vi "myRIO_BRig_FPGA_v3,3.vi"() -> ()   [LabVIEW 2014]
uses:
  <vilib>/rvi/FXPMathLib/FxpDiv/subVIs/nifxpmath_Div_SimConfig.ctl
  <vilib>/rvi/FXPMathLib/FxpSinAndCos/subVIs/nifxpmath_SinAndCos_SimConfig.ctl
  <vilib>/rvi/FXPMathLib/FxpDiv/simVIs/DllFxpDivTemp_sub.vi
  <vilib>/rvi/FXPMathLib/FxpSinAndCos/simVIs/DllFxpSinAndCosTemp_sub.vi
  <vilib>/rvi/Emulation/niFpgaGetClockAttributes.vi
  <vilib>/rvi/Emulation/niFpgaSctlEmulationGetInTimedLoop.vi
  <vilib>/rvi/Emulation/niFpgaEmulationReportErrorSimple.vi
  <vilib>/rvi/eio/common/nirviEmuTemplateMethod_errors.vi
  <vilib>/rvi/Emulation/niFpgaCriticalErrorInLSC.vi
  <vilib>/rvi/FXPMathLib/FxpDiv/XNode/nifxpmath_Div.xnode
  <vilib>/rvi/FXPMathLib/FxpMul/XNode/nifxpmath_Multiplier.xnode
  <vilib>/rvi/FXPMathLib/FxpSinAndCos/XNode/nifxpmath_SinAndCos.xnode
  <vilib>/rvi/FXPMathLib/FxpSub/XNode/nifxpmath_Sub.xnode
  <vilib>/eio/EIONode/EIONode.xnode
  <vilib>/rvi/FXPMathLib/sim/FxpSim.dll
panel:
  in  "laser_Nshutter":u32=100
  in  "AnaOut_0":u16
  in  "f_time_select":u32=173
  in  "laser_Nvalley":u32=100
  in  "laser_Npeak":u32=100
  in  "laserledMTrig":bool
  in  "tCycle_laser_wro":u32=100
  in  "tDelay_laser_wro":u32
  in  "tCycle_laser_rew":u32=100
  in  "tDelay_laser_rew":u32
  in  "laserResponse_reward_LED":bool
  in  "laserResponse_wrong_LED":bool
  out "SelectWrong":bool
  out "SelectReward":bool
  in  "laserResponse_wrong":bool
  in  "laserResponse_reward":bool
  in  "Left(F)_or_Right(T)":bool
  in  "ignoreWrong":bool
  in  "SelectionState":bool
  in  "laserMTrig":bool
  in  "FPGA_Stop":bool
  in  "audioTrigger_L":bool
  in  "audioTrigger_R":bool
  in  "audioFreq_L_Hz":u16=1000 min=1000 max=14000 step=1000
  in  "audioAmp_L":u16=1 min=1 max=32767 step=1
  in  "audioFreq_R_Hz":u16=1000 min=1000 max=14000 step=1000
  in  "audioAmp_R":u16=1 min=1 max=32767 step=1
  in  "A3_SL":bool
  in  "A1_SR":bool
  in  "Counts_Reset":bool
  out "A4_LickR":u32
  out "A2_LickL":u32
  in  "A6_Act":bool
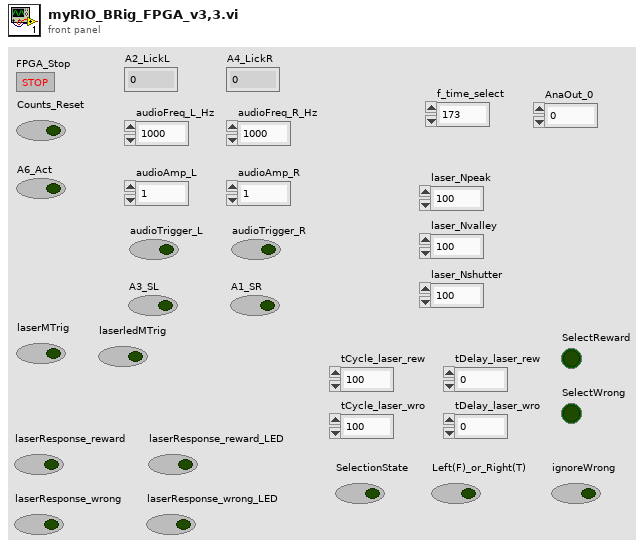
[diagram p1: front panel]
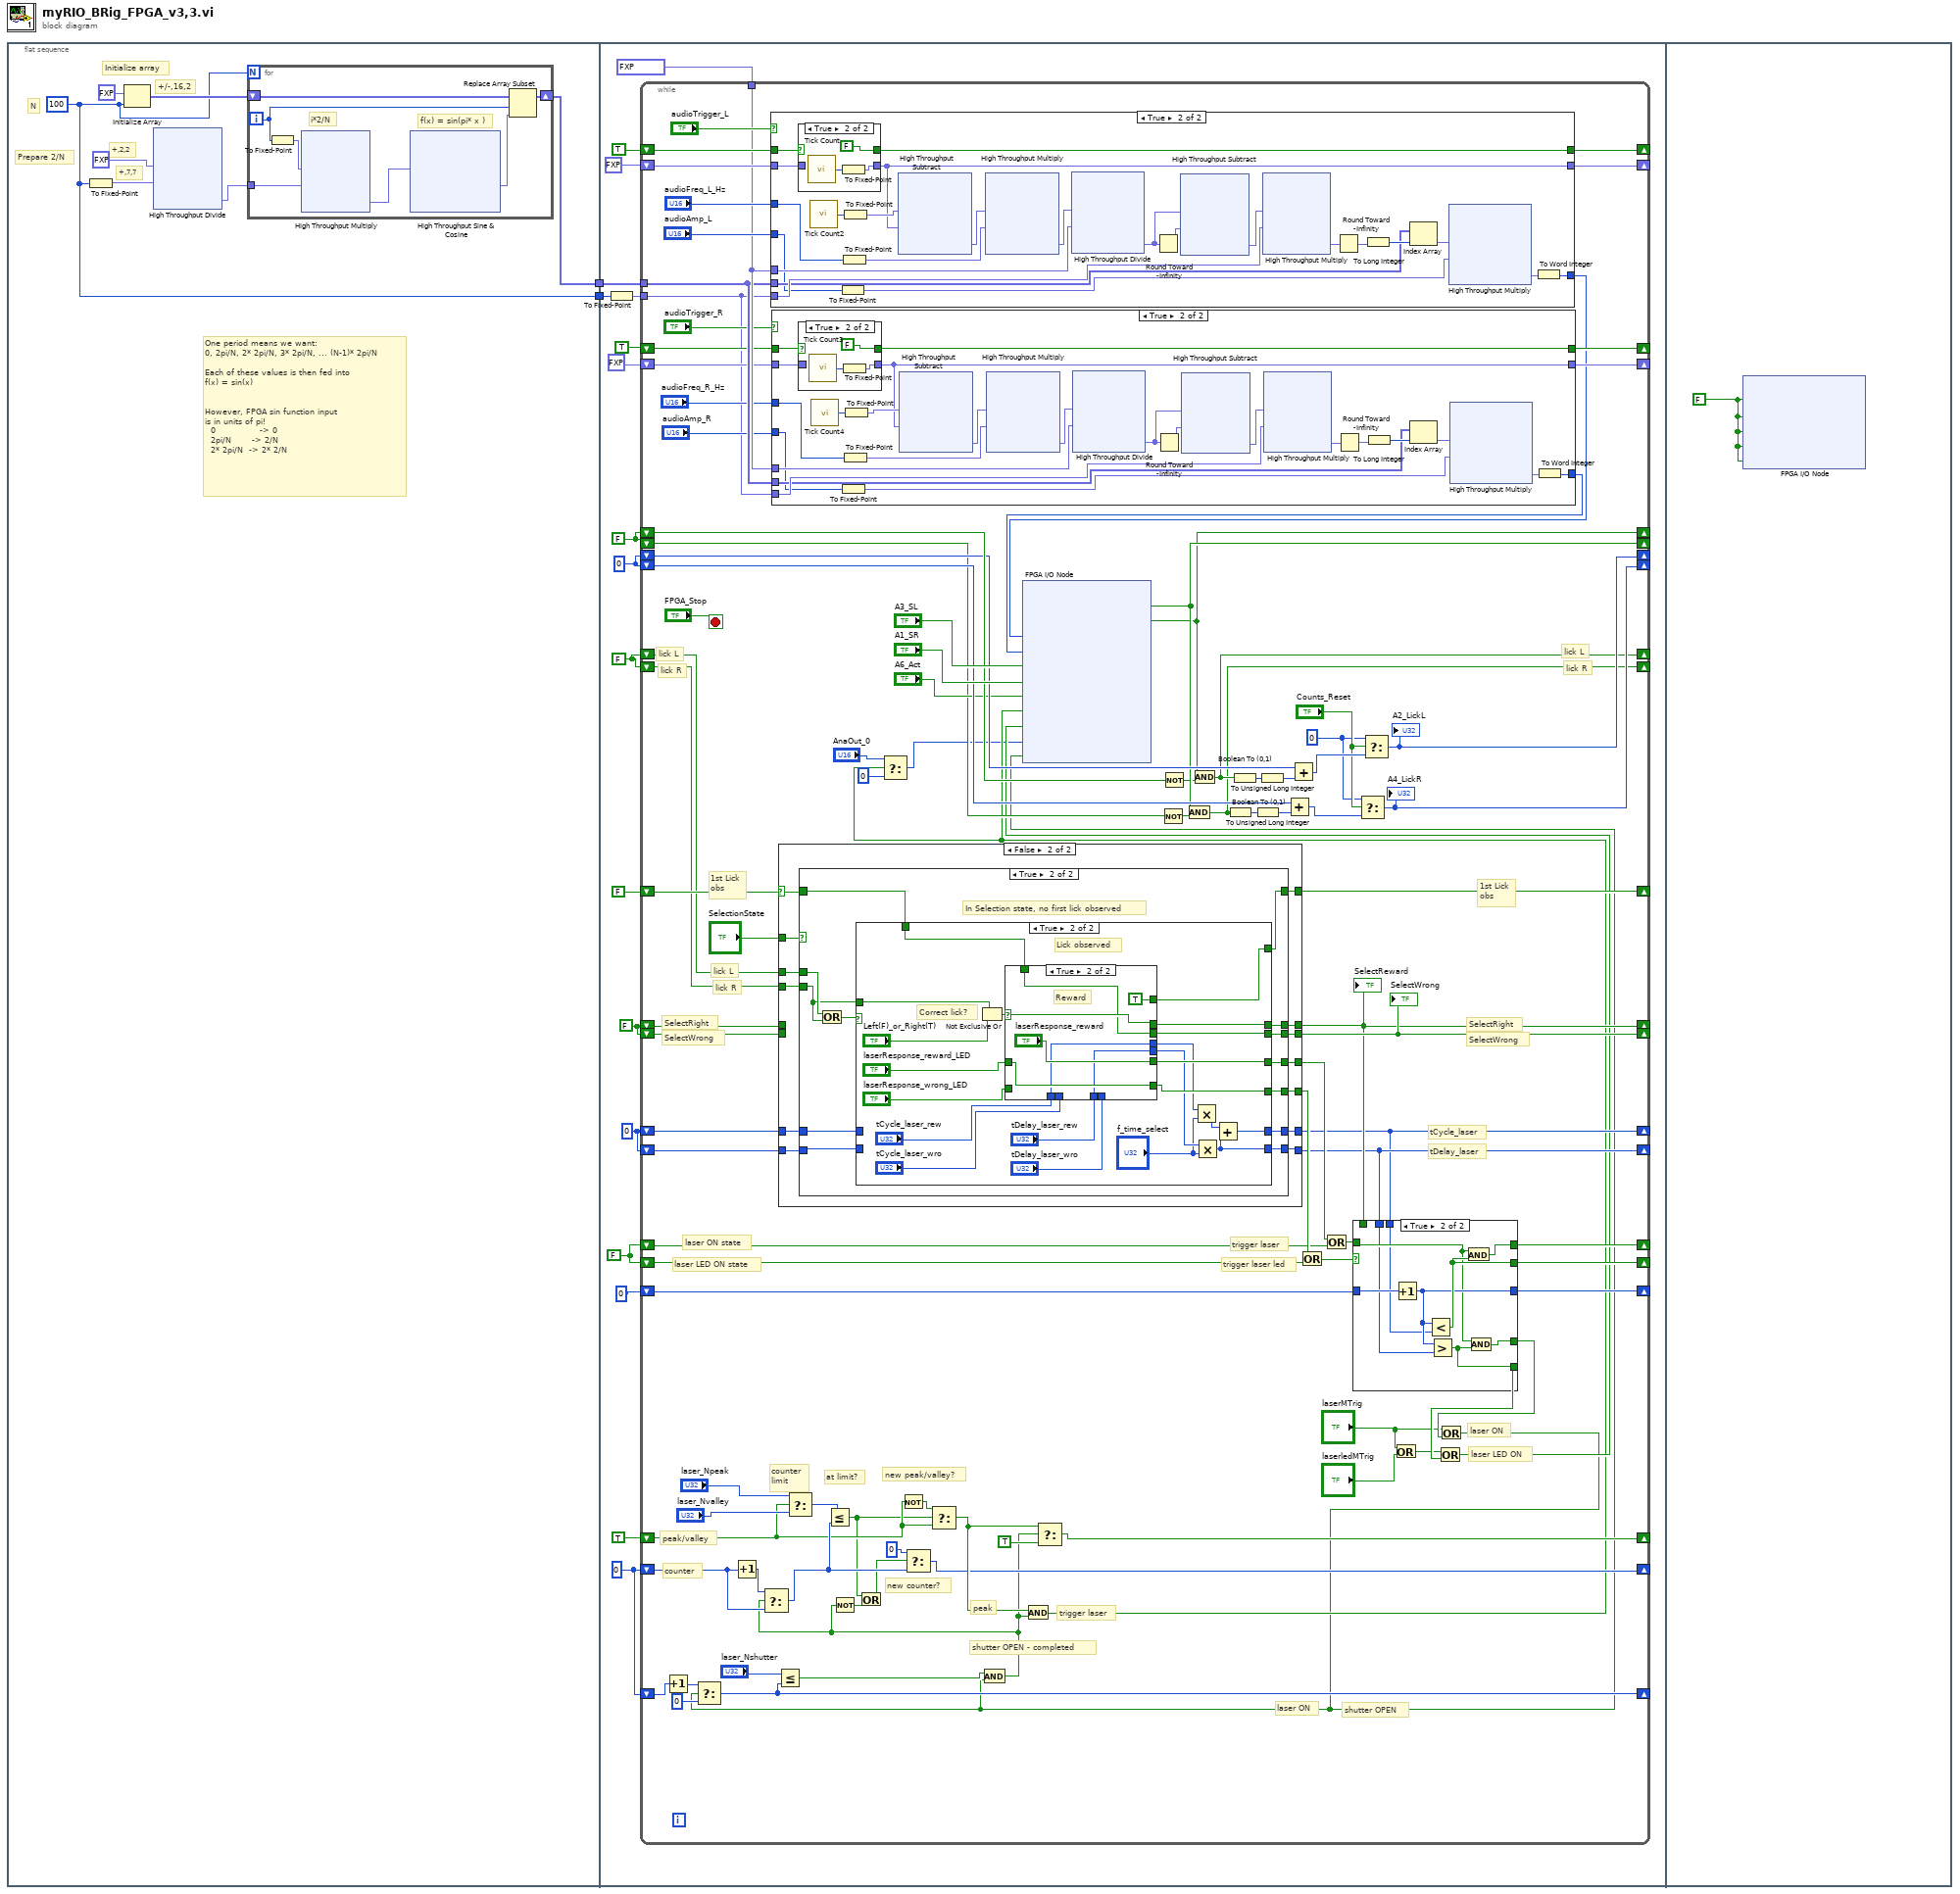
[diagram p0: block diagram]
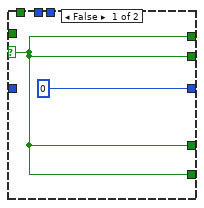
[diagram p2: hidden frame]
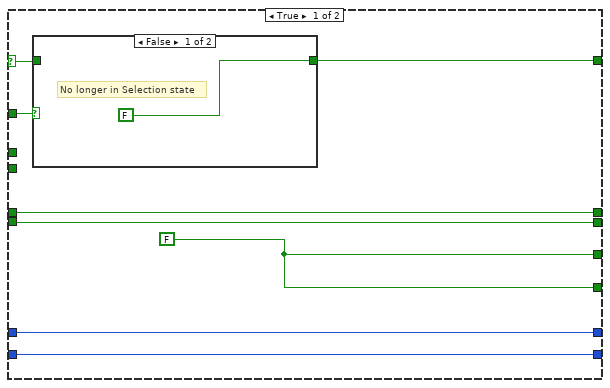
[diagram p3: hidden frame]
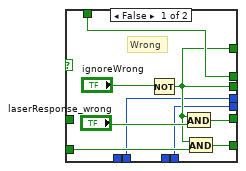
[diagram p7: hidden frame]
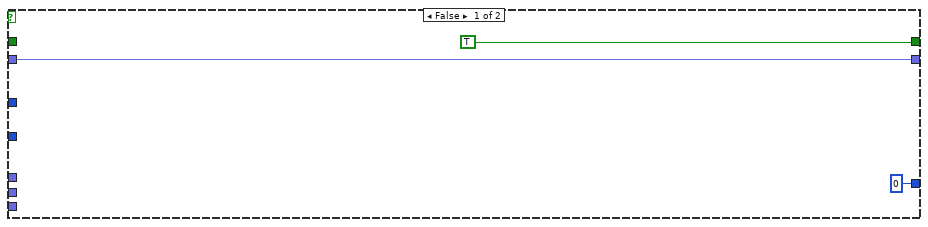
[diagram p8: hidden frame]
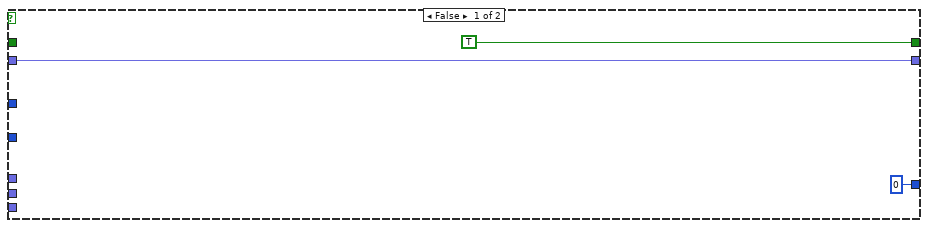
[diagram p10: hidden frame]
diagram:
  n1 = flat-sequence {
    tunnel: [w4] -> w2
    tunnel: [w3] -> w1
    tunnel: w2 -> [w86]
    tunnel: w1 -> [w88]
    frame #0 {
      w3 = 100 ("dimension size")
      # "N"
      # "+,7,7"
      # "+,2,2"
      # "+/-,16,2"
      # "Prepare 2/N"
      # "One period means we want:\n0, 2pi/N, 2* 2pi/N, 3* 2pi/N, ... (N-1)* 2pi/N\n\nEach of these values is then fed into\nf(x) = sin(x)\n\n\nHowever, FPGA sin function input\nis in units of pi!\n  0               -> 0\n  2pi/N       -> 2/N\n  2* 2pi/N  -> 2* 2/N"
      # "Initialize array"
      n2 = To Fixed-Point(number=w3) -> (fixed-point=w6:fxp<+,7,7>)  [unwired: 1 in]
      n3 = Initialize Array(fxp<+/-,16,2> 0.0 ("element"), w3) -> (w9:fxp<+/-,16,2>[])
      n4 = xnode "High Throughput Divide"("x"=fxp<+,2,2> 2.0, "y"=w6) -> ("x/y"=w5:fxp<+,27,0>)
      n5 = for {
        N: w3 -> [_]
        shift-right: [w42] -> w4
        shift-left: w9 -> [w43]
        tunnel: w5 -> [w38]
        i -> [w41]
        # "f(x) = sin(pi* x )"
        # "i*2/N"
        n6 = To Fixed-Point(number=w41) -> (fixed-point=w39:fxp<+,7,7>)  [unwired: 1 in]
        n7 = xnode ("High Throughput Multiply")("x"=w39, "y"=w38) -> ("x*y"=w37:fxp<+,34,7>)
        n8 = xnode "High Throughput Sine & Cosine"("x (pi)"=w37) -> ("sin(x)"=w40:fxp<+/-,16,2>)  [unwired: 1 out]
        n9 = Replace Array Subset(array=w43, new element=w40, index=w41) -> (w42:fxp<+/-,16,2>[])
      }
    }
    frame #1 {
      w74 = u32 0
      w76 = u32 0
      w78 = FALSE
      w77 = FALSE
      w81 = FALSE
      w82 = FALSE
      w83 = u32 0
      n10 = To Fixed-Point(number=w88) -> (fixed-point=w87:fxp<+,7,7>)  [unwired: 1 in]
      n11 = while {
        shift-right: [w185] -> _
        shift-left: TRUE -> [w189]
        shift-right: [w184] -> _
        shift-left: fxp<+,32,32> 0.0 -> [w188]
        tunnel: fxp<+,17,26> 40000000.0 -> [w183]
        tunnel: w87 -> [w176]
        tunnel: w86 -> [w182]
        shift-right: [w175] -> _
        shift-left: TRUE -> [w181]
        shift-right: [w174] -> _
        shift-left: fxp<+,32,32> 0.0 -> [w180]
        shift-right: [w151] -> _
        shift-left: w83 -> [w163]
        shift-right: [w154] -> _
        shift-left: w83 -> [w167]
        shift-right: [w155] -> _
        shift-left: w82 -> [w158]
        shift-right: [w152] -> _
        shift-left: w82 -> [w164]
        shift-right: [w149] -> _
        shift-left: FALSE -> [w148]
        shift-right: [w147] -> _
        shift-left: w81 -> [w145]
        shift-right: [w146] -> _
        shift-left: w81 -> [w144]
        shift-right: [w134] -> _
        shift-left: w77 -> [w136]
        shift-right: [w142] -> _
        shift-left: u32 0 -> [w143]
        shift-right: [w128] -> _
        shift-left: w78 -> [w140]
        shift-right: [w141] -> _
        shift-left: w78 -> [w139]
        shift-right: [w135] -> _
        shift-left: w77 -> [w132]
        shift-right: [w124] -> _
        shift-left: w76 -> [w127]
        shift-right: [w125] -> _
        shift-left: w76 -> [w126]
        shift-right: [w107] -> _
        shift-left: w74 -> [w118]
        shift-right: [w108] -> _
        shift-left: TRUE -> [w111]
        shift-right: [w95] -> _
        shift-left: w74 -> [w99]
        stop <- "FPGA_Stop" stop-if-true
        w160 = u32 0
        # "shutter OPEN"
        # "shutter OPEN - completed"
        # "trigger laser"
        # "peak"
        # "laser ON"
        # "new peak/valley?"
        # "counter"
        # "peak/valley"
        # "new counter?"
        # "at limit?"
        # "counter\nlimit"
        # "tDelay_laser"
        # "tCycle_laser"
        # "laser LED ON"
        # "laser ON"
        # "laser LED ON state"
        # "laser ON state"
        # "SelectWrong"
        # "SelectRight"
        # "SelectWrong"
        # "SelectRight"
        # "lick R"
        # "lick L"
        # "1st Lick\nobs"
        # "1st Lick\nobs"
        # "lick R"
        # "lick L"
        # "lick R"
        # "lick L"
        # "trigger laser led"
        # "trigger laser"
        n12 = Increment(x=w99) -> (x+1=w98:u32)
        n13 = Increment(x=w118) -> (x+1=w116:u32)
        n14 = case shown="True" "audioTrigger_L" {
          tunnel: w189 -> [_ w367]
          tunnel: w188 -> [w343 w366]
          tunnel: "audioFreq_L_Hz" -> [_ w363]
          tunnel: w183 -> [_ w360]
          tunnel: [w343 w344] -> w184
          tunnel: [TRUE w357] -> w185
          tunnel: w176 -> [_ w356]
          tunnel: w182 -> [_ w351]
          tunnel: "audioAmp_L" -> [_ w349]
          tunnel: [i16 0 w346] -> w170
          frame False {
          }
          frame True {
            n15 = case shown="True" w367 {
              selector: w367 -> [w396 _]
              tunnel: [w396 FALSE] -> w357
              tunnel: w366 -> [w395 _]
              tunnel: [w395 w397] -> w344
              frame False {
              }
              frame True {
                n16 = call "Tick Count"() -> ("Tick Count(Ticks)"=w399:u32)
                n17 = To Fixed-Point(number=w399) -> (fixed-point=w397:fxp<+,32,32>)  [unwired: 1 in]
              }
            }
            n18 = call "Tick Count2"() -> ("Tick Count(Ticks)"=w365:u32)
            n19 = To Fixed-Point(number=w349) -> (fixed-point=w348:fxp<+,15,15>)  [unwired: 1 in]
            n20 = To Fixed-Point(number=w363) -> (fixed-point=w362:fxp<+,14,14>)  [unwired: 1 in]
            n21 = To Fixed-Point(number=w365) -> (fixed-point=w345:fxp<+,32,32>)  [unwired: 1 in]
            n22 = xnode "High Throughput Subtract"("x"=w345, "y"=w344) -> ("x-y"=w364:fxp<+,32,32>)
            n23 = xnode ("High Throughput Multiply")("x"=w364, "y"=w362) -> ("x*y"=w361:fxp<+,46,46>)
            n24 = xnode "High Throughput Divide"("x"=w361, "y"=w360) -> ("x/y"=w359:fxp<+,34,21>)
            n25 = Round Toward -Infinity(1:w359) -> (0:w358:fxp<+,21,21>)
            n26 = xnode "High Throughput Subtract"("x"=w359, "y"=w358) -> ("x-y"=w355:fxp<+,14,1>)
            n27 = xnode ("High Throughput Multiply")("x"=w355, "y"=w356) -> ("x*y"=w352:fxp<+,21,8>)
            n28 = Round Toward -Infinity(1:w352) -> (0:w354:fxp<+,8,8>)
            n29 = To Long Integer(number=w354) -> (32bit integer=w353:i32)
            n30 = Index Array(array=w351, index=w353) -> (element=w350:fxp<+/-,16,2>)
            n31 = xnode ("High Throughput Multiply")("x"=w350, "y"=w348) -> ("x*y"=w347:fxp<+/-,31,17>)
            n32 = To Word Integer(number=w347) -> (16bit integer=w346:i16)
          }
        }
        n33 = case shown="True" "audioTrigger_R" {
          tunnel: w181 -> [_ w308]
          tunnel: w180 -> [w284 w307]
          tunnel: "audioFreq_R_Hz" -> [_ w304]
          tunnel: w183 -> [_ w301]
          tunnel: [w284 w285] -> w174
          tunnel: [TRUE w298] -> w175
          tunnel: w176 -> [_ w297]
          tunnel: w182 -> [_ w292]
          tunnel: "audioAmp_R" -> [_ w290]
          tunnel: [i16 0 w287] -> w171
          frame False {
          }
          frame True {
            n34 = case shown="True" w308 {
              selector: w308 -> [w337 _]
              tunnel: [w337 FALSE] -> w298
              tunnel: w307 -> [w336 _]
              tunnel: [w336 w338] -> w285
              frame False {
              }
              frame True {
                n35 = call "Tick Count3"() -> ("Tick Count(Ticks)"=w340:u32)
                n36 = To Fixed-Point(number=w340) -> (fixed-point=w338:fxp<+,32,32>)  [unwired: 1 in]
              }
            }
            n37 = call "Tick Count4"() -> ("Tick Count(Ticks)"=w306:u32)
            n38 = To Fixed-Point(number=w290) -> (fixed-point=w289:fxp<+,15,15>)  [unwired: 1 in]
            n39 = To Fixed-Point(number=w304) -> (fixed-point=w303:fxp<+,14,14>)  [unwired: 1 in]
            n40 = To Fixed-Point(number=w306) -> (fixed-point=w286:fxp<+,32,32>)  [unwired: 1 in]
            n41 = xnode "High Throughput Subtract"("x"=w286, "y"=w285) -> ("x-y"=w305:fxp<+,32,32>)
            n42 = xnode ("High Throughput Multiply")("x"=w305, "y"=w303) -> ("x*y"=w302:fxp<+,46,46>)
            n43 = xnode "High Throughput Divide"("x"=w302, "y"=w301) -> ("x/y"=w300:fxp<+,34,21>)
            n44 = Round Toward -Infinity(1:w300) -> (0:w299:fxp<+,21,21>)
            n45 = xnode "High Throughput Subtract"("x"=w300, "y"=w299) -> ("x-y"=w296:fxp<+,14,1>)
            n46 = xnode ("High Throughput Multiply")("x"=w296, "y"=w297) -> ("x*y"=w293:fxp<+,21,8>)
            n47 = Round Toward -Infinity(1:w293) -> (0:w295:fxp<+,8,8>)
            n48 = To Long Integer(number=w295) -> (32bit integer=w294:i32)
            n49 = Index Array(array=w292, index=w294) -> (element=w291:fxp<+/-,16,2>)
            n50 = xnode ("High Throughput Multiply")("x"=w291, "y"=w289) -> ("x*y"=w288:fxp<+/-,31,17>)
            n51 = To Word Integer(number=w288) -> (16bit integer=w287:i16)
          }
        }
        n52 = case shown="False" w148 {
          selector: w148 -> [w208 w223]
          tunnel: "SelectionState" -> [w210 w225]
          tunnel: [w209 w224] -> w149
          tunnel: w145 -> [_ w222]
          tunnel: w144 -> [_ w221]
          tunnel: [w207 w220] -> w133
          tunnel: [w205 w219] -> w128
          tunnel: [w206 w218] -> w141
          tunnel: w140 -> [w205 _]
          tunnel: w139 -> [w206 _]
          tunnel: [w207 w217] -> w137
          tunnel: [w204 w216] -> w124
          tunnel: [w203 w215] -> w125
          tunnel: w127 -> [w204 w214]
          tunnel: w126 -> [w203 w213]
          frame True {
            w207 = FALSE
            n53 = case shown="False" w210 {
              tunnel: [FALSE w212] -> w209
              tunnel: w208 -> [_ w212]
              frame False {
                # "No longer in Selection state"
              }
              frame True {
                # "Already observed first lick, no other action"
              }
            }
          }
          frame False {
            n54 = case shown="True" w225 {
              tunnel: [w228 w238] -> w224
              tunnel: w223 -> [w228 w234]
              tunnel: w222 -> [_ w240]
              tunnel: w221 -> [_ w239]
              tunnel: [w228 w237] -> w220
              tunnel: [w228 w236] -> w219
              tunnel: [w228 w235] -> w218
              tunnel: [w228 w233] -> w217
              tunnel: [w227 w232] -> w216
              tunnel: [w226 w231] -> w215
              tunnel: w214 -> [w227 w230]
              tunnel: w213 -> [w226 w229]
              frame False {
                # "Not in Selection state"
              }
              frame True {
                # "In Selection state, no first lick observed"
                n55 = Or(x=w240, y=w239) -> (x .or. y?=w241:bool)
                n56 = case shown="True" w241 {
                  tunnel: w239 -> [_ w264]
                  tunnel: [w244 w257] -> w238
                  tunnel: [w244 w262] -> w237
                  tunnel: [w244 w261] -> w236
                  tunnel: [w244 w260] -> w235
                  tunnel: w234 -> [w244 w259]
                  tunnel: [w244 w258] -> w233
                  tunnel: [w243 w246] -> w232
                  tunnel: [w242 w245] -> w231
                  tunnel: w230 -> [w243 _]
                  tunnel: w229 -> [w242 _]
                  frame False {
                  }
                  frame True {
                    # "Correct lick?"
                    # "Lick observed"
                    n57 = Not Exclusive Or(1:"Left(F)_or_Right(T)", 2:w264) -> (0:w263:bool)
                    n58 = case shown="True" w263 {
                      selector: w263 -> [_ w280]
                      tunnel: [w271 "laserResponse_reward"] -> w262
                      tunnel: [w269 w276] -> w260
                      tunnel: [w273 w280] -> w261
                      tunnel: w259 -> [w273 w276]
                      tunnel: [w270 w278] -> w258
                      tunnel: [w269 TRUE] -> w257
                      tunnel: "laserResponse_reward_LED" -> [_ w278]
                      tunnel: "laserResponse_wrong_LED" -> [w268 _]
                      tunnel: "tCycle_laser_rew" -> [_ w275]
                      tunnel: "tCycle_laser_wro" -> [w266 _]
                      tunnel: "tDelay_laser_rew" -> [_ w277]
                      tunnel: "tDelay_laser_wro" -> [w267 _]
                      tunnel: [w267 w277] -> w249
                      tunnel: [w266 w275] -> w248
                      frame False {
                        # "Wrong"
                        n59 = Not(x="ignoreWrong") -> (.not. x?=w269:bool)
                        n60 = And(x=w269, y="laserResponse_wrong") -> (x .and. y?=w271:bool)
                        n61 = And(x=w269, y=w268) -> (x .and. y?=w270:bool)
                      }
                      frame True {
                        # "Reward"
                      }
                    }
                    n62 = Multiply(x=w248, y="f_time_select") -> (x*y=w250:u32)
                    n63 = Multiply(x=w249, y="f_time_select") -> (x*y=w245:u32)
                    n64 = Add(x=w250, y=w245) -> (x+y=w246:u32)
                  }
                }
              }
            }
          }
        }
        "SelectWrong" <- w141
        "SelectReward" <- w128
        n65 = Select(t="laser_Npeak", s=w111, f="laser_Nvalley") -> (s? t:f=w120:u32)
        n66 = Not(x=w111) -> (.not. x?=w112:bool)
        n67 = Not(x=w158) -> (.not. x?=w157:bool)
        n68 = Not(x=w164) -> (.not. x?=w153:bool)
        n69 = Or(x=w137, y=w136) -> (x .or. y?=w138:bool)
        n70 = Or(x=w133, y=w132) -> (x .or. y?=w131:bool)
        n71 = case shown="True" w138 {
          selector: w138 -> [w192 _]
          tunnel: w143 -> [_ w202]
          tunnel: [u32 0 w199] -> w142
          tunnel: [w192 w200] -> w134
          tunnel: [w192 w201] -> w135
          tunnel: w131 -> [_ w198]
          tunnel: [w192 w197] -> w129
          tunnel: [w192 w196] -> w130
          tunnel: w128 -> [_ _]
          tunnel: w125 -> [_ w195]
          tunnel: w124 -> [_ w194]
          frame False {
          }
          frame True {
            n72 = Increment(x=w202) -> (x+1=w199:u32)
            n73 = Less?(x=w199, y=w194) -> (x < y?=w200:bool)
            n74 = Greater?(x=w199, y=w195) -> (0:w197:bool)
            n75 = And(x=w198, y=w200) -> (x .and. y?=w201:bool)
            n76 = And(x=w198, y=w197) -> (x .and. y?=w196:bool)
          }
        }
        n77 = Or(x="laserMTrig", y="laserledMTrig") -> (x .or. y?=w122:bool)
        n78 = Or(x=w122, y=w129) -> (x .or. y?=w117:bool)
        n79 = Or(x="laserMTrig", y=w130) -> (x .or. y?=w92:bool)
        n80 = Select(t=w98, s=w92, f=u32 0) -> (s? t:f=w95:u32)
        n81 = Less Or Equal?(x="laser_Nshutter", y=w95) -> (x <= y?=w94:bool)
        n82 = And(x=w94, y=w92) -> (x .and. y?=w93:bool)
        n83 = Select(t=w116, s=w93, f=w118) -> (s? t:f=w115:u32)
        n84 = Less Or Equal?(x=w120, y=w115) -> (x <= y?=w105:bool)
        n85 = Not(x=w93) -> (.not. x?=w106:bool)
        n86 = Or(x=w105, y=w106) -> (x .or. y?=w104:bool)
        n87 = Select(t=u32 0, s=w104, f=w115) -> (s? t:f=w107:u32)
        n88 = Select(t=w112, s=w105, f=w111) -> (s? t:f=w110:bool)
        n89 = And(x=w110, y=w93) -> (x .and. y?=w103:bool)
        n90 = Select(t="AnaOut_0", s=w103, f=u16 0) -> (s? t:f=w102:u16)
        n91 = xnode "FPGA I/O Node"("AudioOut/Left"=w170, "AudioOut/Right"=w171, "ConnectorA/DIO3"="A3_SL", "ConnectorA/DIO1"="A1_SR", "ConnectorA/DIO7"="A6_Act", "ConnectorA/DIO0"=w103, "ConnectorA/DIO14"=w117, "ConnectorB/AO0"=w102, "ConnectorA/DIO6"=w92) -> ("ConnectorA/DIO4"=w155:bool, "ConnectorA/DIO2"=w152:bool)  [unwired: 11 in, 11 out]
        n92 = Select(t=w110, s=w93, f=TRUE) -> (s? t:f=w108:bool)
        n93 = And(x=w155, y=w157) -> (x .and. y?=w146:bool)
        n94 = And(x=w152, y=w153) -> (x .and. y?=w147:bool)
        n95 = Boolean To (0,1)(Boolean=w146) -> (0, 1=w169:i16)
        n96 = Boolean To (0,1)(Boolean=w147) -> (0, 1=w166:i16)
        n97 = To Unsigned Long Integer(number=w169) -> (unsigned 32bit integer=w168:u32)
        n98 = To Unsigned Long Integer(number=w166) -> (unsigned 32bit integer=w165:u32)
        n99 = Add(x=w167, y=w168) -> (x+y=w156:u32)
        n100 = Add(x=w163, y=w165) -> (x+y=w162:u32)
        n101 = Select(t=w160, s="Counts_Reset", f=w156) -> (s? t:f=w154:u32)
        "A4_LickR" <- w154
        n102 = Select(t=w160, s="Counts_Reset", f=w162) -> (s? t:f=w151:u32)
        "A2_LickL" <- w151
      }
    }
    frame #2 {
      w400 = FALSE ("ConnectorA/DIO3")
      n103 = xnode "FPGA I/O Node"("ConnectorC/DIO3"=w400, "ConnectorC/DIO1"=w400, "ConnectorC/DIO0"=w400, "ConnectorC/DIO6"=w400, "ConnectorC/DIO7"=w400) -> ()  [unwired: 5 in, 5 out]
    }
  }
